vi "Logging Message Loop.vi"(8 "error in (no error)":errorcluster, 11 "Message Queues":T5) -> (0 "error out":errorcluster)   [LabVIEW 2018, in "Logging.lvlib"]
doc: "The message loop subVI to handle messages pertaining to logging data."
uses:
  Logging.lvlib
  Support/Message Queue/All Message Queues.ctl
  Support/Message Queue/Message Cluster.ctl
  Controls/Data Queue.ctl
  Controls/Acquired Data.ctl
  Controls/Data Notifier.ctl
  Settings/Settings.ctl
  Acquisition/Hardware Configuration.ctl
  Logging Configuration.ctl
  <vilib>/addons/database/Connection.llb/Conn ObjectReference.ctl
  Controls/Location Ring.ctl
  Controls/Time Remaining.ctl
  Logging State.ctl
  Support/Message Queue/Enqueue Message (Single).vi
  <vilib>/Utility/error.llb/Error Cluster From Error Code.vi
  <vilib>/ErrorRing/Error Ring.xnode
  support/Message Queue/Message Queue.lvlib
  <vilib>/addons/database/NI_Database_API.lvlib
  Acquisition/Acquisition.lvlib
  Settings/Settings.lvlib
panel:
  in  "C&C Data In":T1={"Hardware Configuration"={"COM Port"="", "Reference Distance"=0.0, "Sensor SN"=""}, "Logging Configuration"={"Log File Base Path"=path "", "Datafile Ref"=refnum, "Database Ref"=refnum}, "UI Refs"={"Start Ref"=refnum, "Settings Ref"=refnum, "Stop Ref"=refnum, "Exit Ref"=refnum, "Status Ref"=refnum, "Data Ref"=refnum, "StatusBox Ref"=refnum, "Location Ref"=refnum, "Operator Ref"=refnum, "Time Ref"=refnum, "Test in Progess Ref"=refnum}, "Calibration Data"={"calibrationID"=0, "operatorID"=0, "sensorID"=0, "start_time"="", "end_time"="", "offset"=0.0, "offset_units"="", "ring_time"=0.0, "error"=0.0, "Passed"=0, "data_storage_location"="", "comments"=""}, "Time Elapsed"=0, "Samples Required"=480} {"Hardware Configuration"."Reference Distance" format="%.3g"}
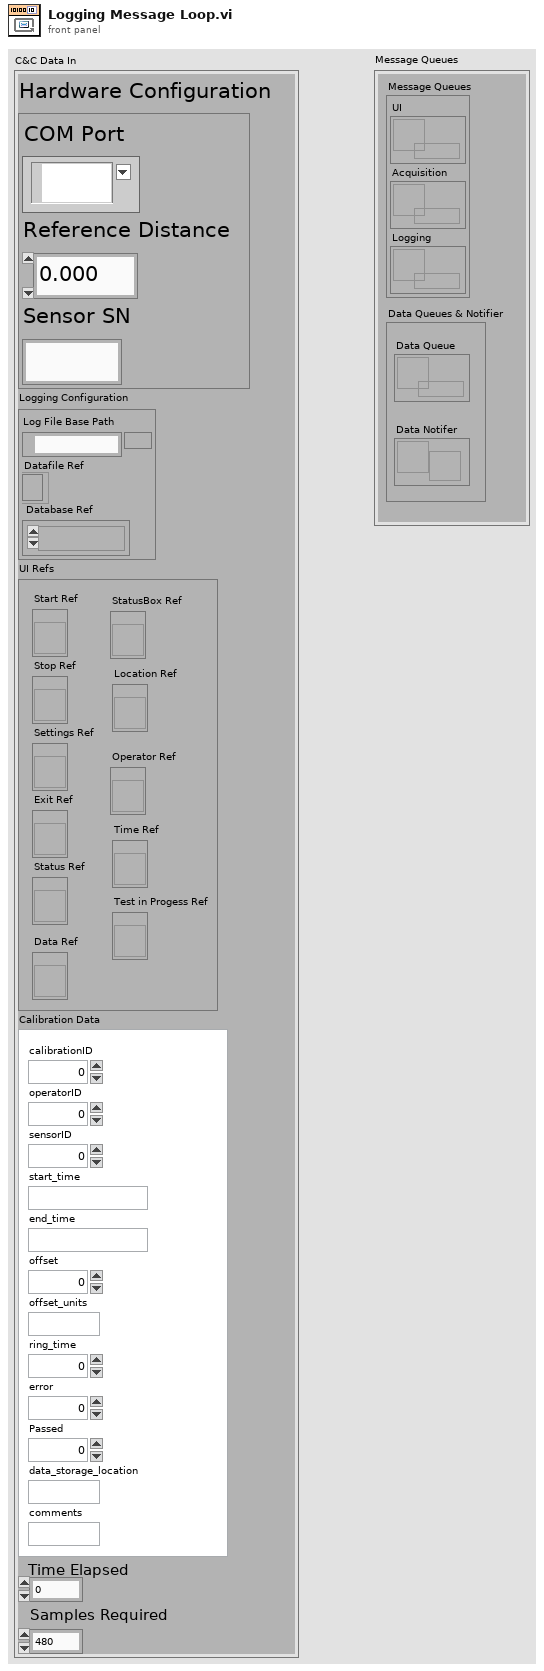
[diagram p1: front panel]
types:
  T1 = typedef "Settings.lvlib/Settings.ctl" = cluster{"Hardware Configuration":T2, "Logging Configuration":T3, "UI Refs":cluster{"Start Ref":refnum<vi>, "Settings Ref":refnum<vi>, "Stop Ref":refnum<vi>, "Exit Ref":refnum<vi>, "Status Ref":refnum<vi>, "Data Ref":refnum<vi>, "StatusBox Ref":refnum<vi>, "Location Ref":refnum<vi>, "Operator Ref":refnum<vi>, "Time Ref":refnum<vi>, "Test in Progess Ref":refnum<vi>}, "Calibration Data":cluster{"calibrationID":u16, "operatorID":u16, "sensorID":u16, "start_time":string, "end_time":string, "offset":dbl, "offset_units":string, "ring_time":dbl, "error":dbl, "Passed":u8, "data_storage_location":string, "comments":string}, "Time Elapsed":u16, "Samples Required":u16}
  T2 = typedef "Acquisition.lvlib/Hardware Configuration.ctl" = cluster{"COM Port":refnum<visa-resource-name>, "Reference Distance":dbl, "Sensor SN":string}
  T3 = typedef "Logging.lvlib/Logging Configuration.ctl" = cluster{"Log File Base Path":path, "Datafile Ref":refnum<file>, "Database Ref":T4}
  T4 = typedef "NI_Database_API.lvlib/Conn ObjectReference.ctl" = refnum<k1>
  T5 = typedef "Message Queue.lvlib/All Message Queues.ctl" = cluster{"Message Queues":cluster{"UI":refnum<queue>, "Acquisition":refnum<queue>, "Logging":refnum<queue>}, "Data Queues & Notifier":cluster{"Data Queue":T6, "Data Notifer":T7}}
  T6 = typedef "Data Queue.ctl" = refnum<queue>
  T7 = typedef "Data Notifier.ctl" = refnum<notifier>
  T8 = enum16{"open", "replace", "create", "open or create", "replace or create", "replace or create with confirmation"}
  T9 = typedef "Logging.lvlib/Logging State.ctl" = enum16{"Idle", "Logging"}
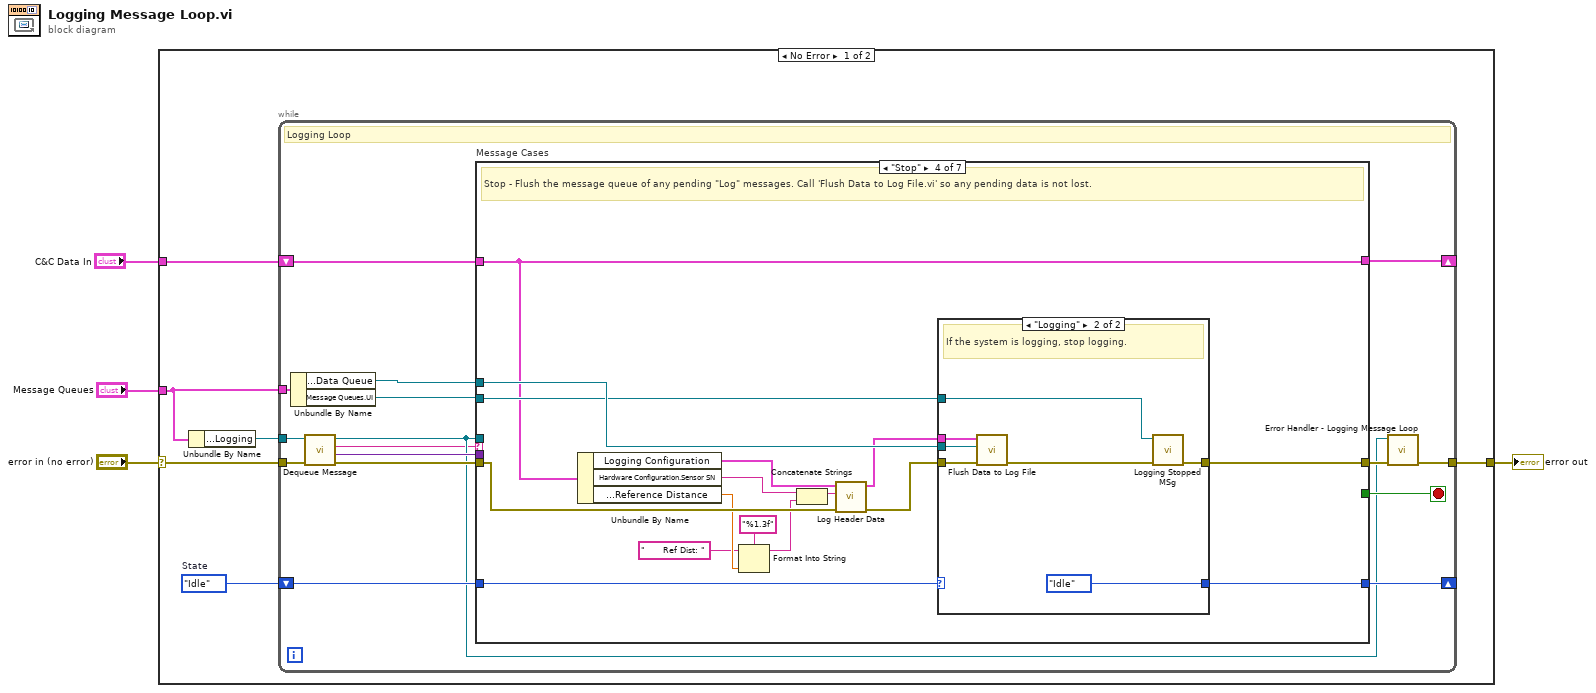
[diagram p0: block diagram]
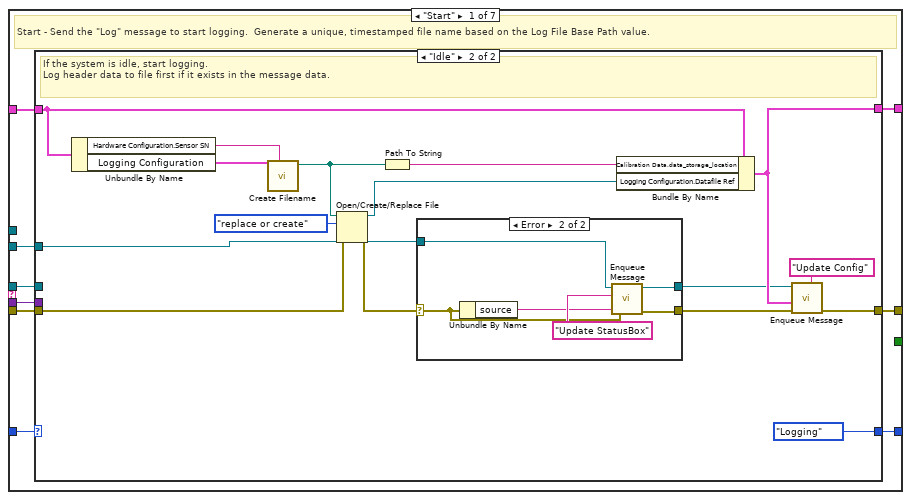
[diagram p2: hidden frame]
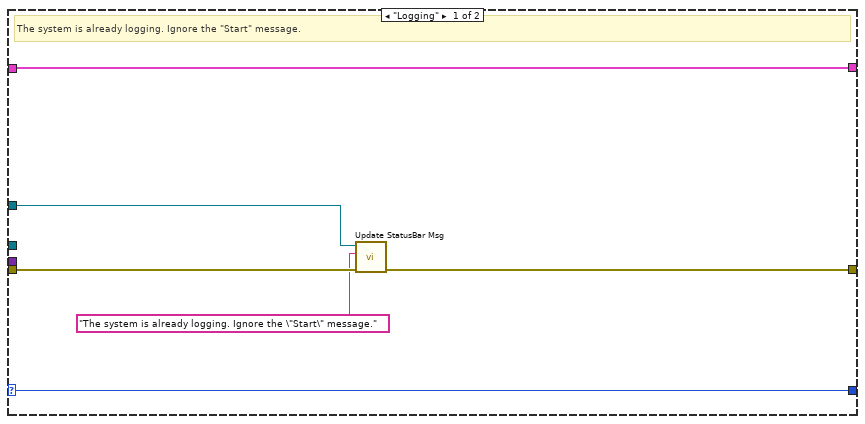
[diagram p3: hidden frame]
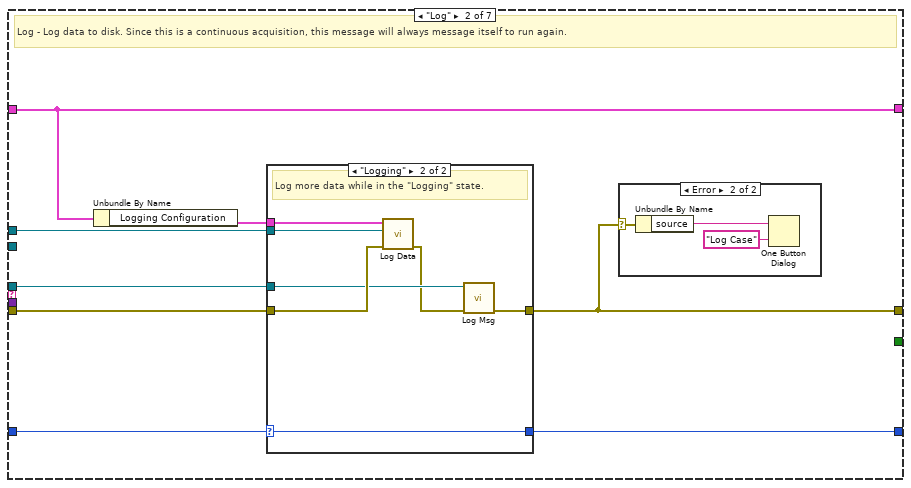
[diagram p5: hidden frame]
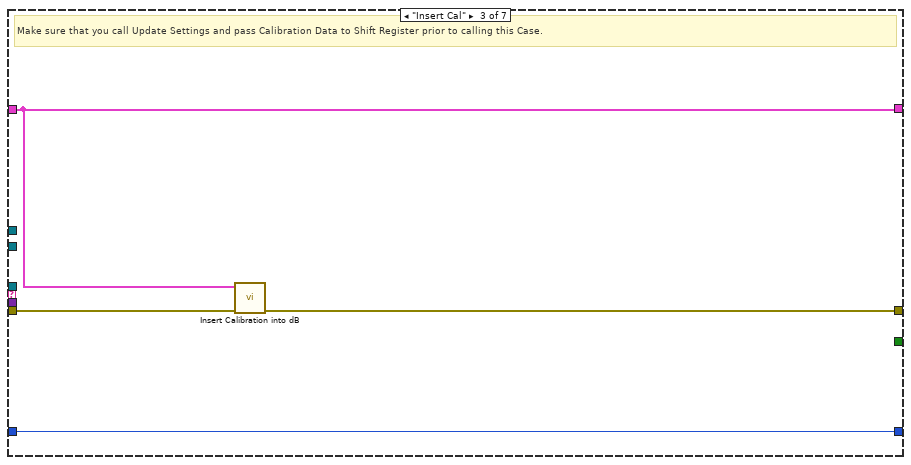
[diagram p8: hidden frame]
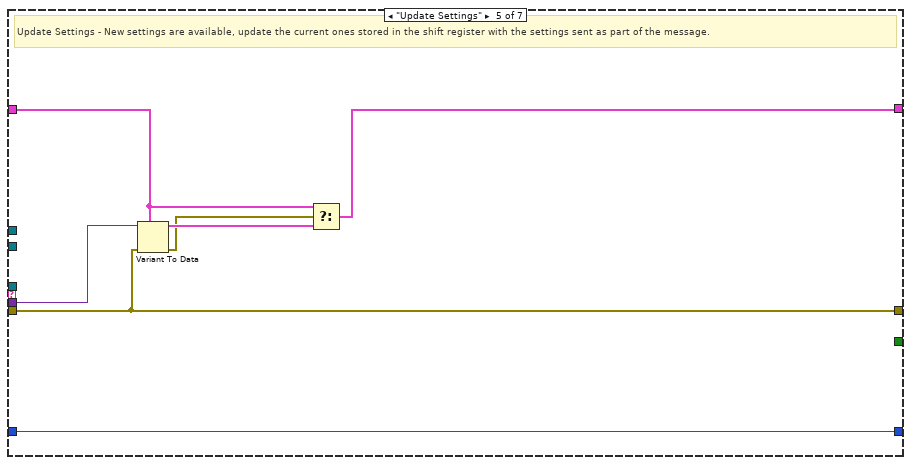
[diagram p10: hidden frame]
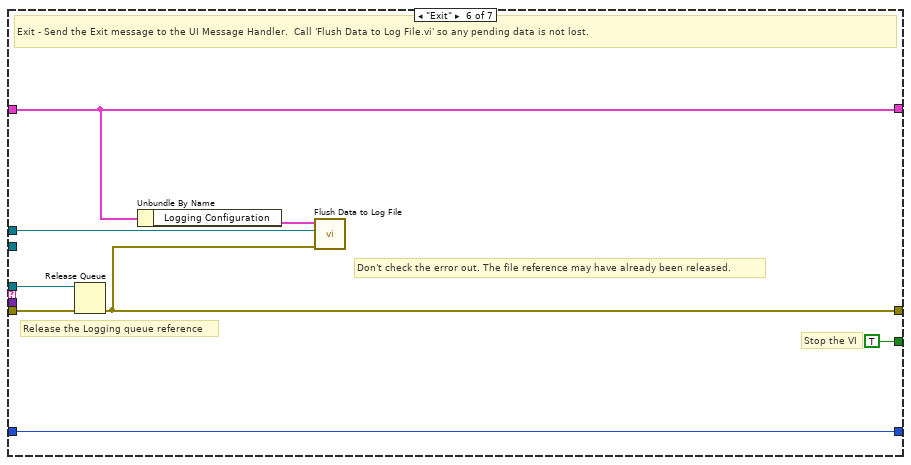
[diagram p11: hidden frame]
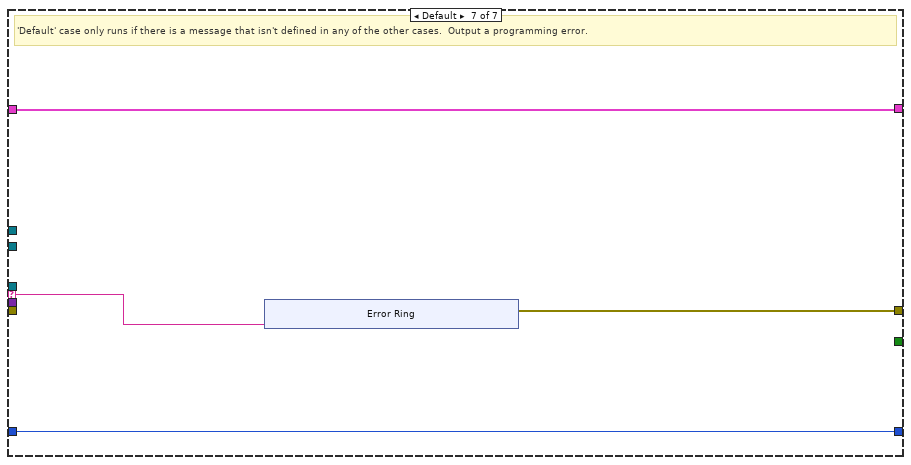
[diagram p12: hidden frame]
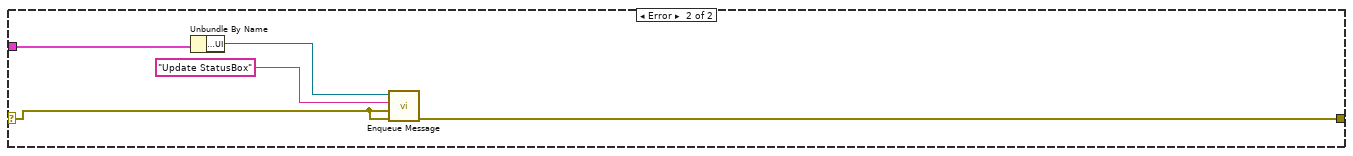
[diagram p13: hidden frame]
diagram:
  n1 = case shown="No Error" "error in (no error)" {
    selector: "error in (no error)" -> [w8 w141]
    tunnel: "Message Queues" -> [w6 w145]
    tunnel: [w9 w142] -> w3
    tunnel: "C&C Data In" -> [w5 _]
    frame No Error {
      w7 = Logging_State."Idle"  # State
      n2 = Unbundle By Name(w6) -> ("Message Queues.Logging"=w10:refnum<queue>)
      n3 = while {
        tunnel: w10 -> [w15]
        shift-right: [w21] -> _
        shift-left: w7 -> [w22]
        tunnel: w8 -> [w25]
        tunnel: [w20] -> w9
        tunnel: w6 -> [w18]
        shift-right: [w11] -> _
        shift-left: w5 -> [w12]
        stop <- w26 stop-if-true
        # "Logging Loop"
        n4 = Unbundle By Name(w18) -> ("Data Queues & Notifier.Data Queue"=w17:T6, "Message Queues.UI"=w16:refnum<queue>)
        n5 = call "Dequeue Message.vi"("error in (no error)"=w25, "Message Queue"=w15) -> ("error out"=w24:errorcluster, "Message Data"=w23:variant, "Message"=w13:string, "dup Message Queue"=w14:refnum<queue>)  [unwired: 6 in]
        n6 = case "Message Cases" shown="\"Stop\"" w13 {
          selector: w13 -> [_ _ _ _ _ _ w131]
          tunnel: w14 -> [w34 w73 _ _ _ w127 _]
          tunnel: w24 -> [w33 w72 w88 w96 w119 w128 _]
          tunnel: [w35 w66 w87 w105 w119 w126 w132] -> w19
          tunnel: [_ _ _ _ _ TRUE _] -> w26
          tunnel: w23 -> [w30 _ _ _ w121 _ _]
          tunnel: w16 -> [w29 _ _ w101 _ _ _]
          tunnel: w17 -> [_ w69 _ w104 _ w125 _]
          tunnel: w22 -> [w32 w71 w89 w103 w118 w124 w133]
          tunnel: [w31 w70 w89 w102 w118 w124 w133] -> w21
          tunnel: w12 -> [w28 w68 w86 w100 w117 w123 w130]
          tunnel: [w27 w68 w86 w100 w116 w123 w130] -> w11
          frame "Start" {
            # "Start - Send the \"Log\" message to start logging.  Generate a unique, timestamped file name based on the Log File Base Path value."
            n7 = case shown="\"Idle\"" w32 {
              selector: w32 -> [w41 _]
              tunnel: [w37 w48] -> w35
              tunnel: w34 -> [_ _]
              tunnel: w33 -> [w38 w55]
              tunnel: [w41 Logging_State."Logging" ("State")] -> w31
              tunnel: w30 -> [_ _]
              tunnel: w29 -> [w39 w47]
              tunnel: w28 -> [w40 w50]
              tunnel: [w40 w51] -> w27
              frame "Logging" {
                # "The system is already logging. Ignore the \"Start\" message."
                n8 = call "Update StatusBar Msg.vi"("error in (no error)"=w38, "Ready..."="The system is already logging. Ignore the \"Start\" message.", "Queue in"=w39) -> ("error out"=w37:errorcluster)  [unwired: 7 in, 1 out]
              }
              frame "Idle" {
                # "If the system is idle, start logging. \nLog header data to file first if it exists in the message data."
                n9 = Unbundle By Name(w50) -> ("Hardware Configuration.Sensor SN"=w42:string, "Logging Configuration"=w49:T3)
                n10 = call "Create Filename.vi"("Sensor SN"=w42, "Logging Configuration"=w49) -> ("appended path"=w53:path)  [unwired: 9 in]
                n11 = Open/Create/Replace File(file path (use dialog)=w53, error in=w55, operation (0:open)=T8."replace or create") -> (refnum out=w54:refnum<file>, error out=w45:errorcluster)  [unwired: 3 in, 1 out]
                n12 = Path To String(path=w53) -> (string=w43:string)
                n13 = case shown="Error" w45 {
                  selector: w45 -> [w59 w60]
                  tunnel: w47 -> [w58 w64]
                  tunnel: [w58 w63] -> w46
                  tunnel: [w59 w62] -> w44
                  frame No Error {
                  }
                  frame Error {
                    n14 = Unbundle By Name(w60) -> ("source"=w61:string)
                    n15 = call-poly "Enqueue Message.vi"("error in (no error)"=w60, "Message Data"=w61, "Message"="Update StatusBox", "Message Queue"=w64) -> ("error out"=w62:errorcluster, "dup Message Queue"=w63:refnum<queue>)  [unwired: 6 in]
                  }
                }
                n16 = Bundle By Name(cluster=w50, "Calibration Data.data_storage_location"=w43, "Logging Configuration.Datafile Ref"=w54) -> (w51:T1)
                n17 = call-poly "Enqueue Message.vi"("error in (no error)"=w44, "Message Data"=w51, "Message"="Update Config", "Message Queue"=w46) -> ("error out"=w48:errorcluster)  [unwired: 6 in, 1 out]
              }
            }
          }
          frame "Log" {
            # "Log - Log data to disk. Since this is a continuous acquisition, this message will always message itself to run again."
            n18 = Unbundle By Name(w68) -> ("Logging Configuration"=w67:T3)
            n19 = case shown="\"Logging\"" w71 {
              selector: w71 -> [w78 w84]
              tunnel: [w77 w79] -> w66
              tunnel: w73 -> [_ w81]
              tunnel: w69 -> [_ w85]
              tunnel: w72 -> [w77 w83]
              tunnel: w67 -> [_ w82]
              tunnel: [w78 w84] -> w70
              frame "Idle" {
                # "Ignore \"Log\" messages when the logging is idle."
              }
              frame "Logging" {
                # "Log more data while in the \"Logging\" state."
                n20 = call "Log Data.vi"("error in (no error)"=w83, "Data Queue"=w85, "Logging Configuration"=w82) -> ("error out"=w80:errorcluster)  [unwired: 8 in]
                n21 = call "Log Msg.vi"("error in (no error)"=w80, "Queue in"=w81) -> ("error out"=w79:errorcluster)  [unwired: 9 in]
              }
            }
            n22 = case shown="Error" w66 {
              selector: w66 -> [_ w75]
              frame No Error {
              }
              frame Error {
                n23 = Unbundle By Name(w75) -> ("source"=w76:string)
                n24 = One Button Dialog(message=w76, button name ("OK")="Log Case") -> ()  [unwired: 1 out]
              }
            }
          }
          frame "Insert Cal" {
            # "Make sure that you call Update Settings and pass Calibration Data to Shift Register prior to calling this Case."
            n25 = call "Insert Calibration into dB.vi"("error in (no error)"=w88, "C&C Data In"=w86) -> ("error out"=w87:errorcluster)  [unwired: 9 in]
          }
          frame "Stop" {
            # "Stop - Flush the message queue of any pending \"Log\" messages. Call 'Flush Data to Log File.vi' so any pending data is not lost."
            n26 = Unbundle By Name(w100) -> ("Logging Configuration"=w99:T3, "Hardware Configuration.Sensor SN"=w95:string, "Hardware Configuration.Reference Distance"=w94:dbl)
            n27 = Format Into String(format string="%1.3f", initial string="      Ref Dist: " ("format string"), w94) -> (resulting string=w91:string)  [unwired: 1 in, 1 out]
            n28 = Concatenate Strings(w95, w91) -> (w93:string)
            n29 = call "Log Header Data.vi"("error in (no error)"=w96, "Header Data"=w93, "Logging Configuration in"=w99) -> ("error out"=w97:errorcluster, "Logging Configuration out"=w98:T3)  [unwired: 7 in]
            n30 = case shown="\"Logging\"" w103 {
              selector: w103 -> [w106 _]
              tunnel: [w107 w110] -> w105
              tunnel: w104 -> [_ w113]
              tunnel: w97 -> [w107 w112]
              tunnel: [w106 Logging_State."Idle" ("State")] -> w102
              tunnel: w101 -> [_ w109]
              tunnel: w98 -> [_ w108]
              frame "Idle" {
                # "The system is already idle. Ignore the \"Stop\" message."
              }
              frame "Logging" {
                # "If the system is logging, stop logging."
                n31 = call "Flush Data to Log File.vi"("error in (no error)"=w112, "Data Queue"=w113, "Logging Configuration"=w108) -> ("error out"=w114:errorcluster)  [unwired: 8 in]
                n32 = call "Logging Stopped MSg.vi"("error in (no error)"=w114, "Queue in"=w109) -> ("error out"=w110:errorcluster)  [unwired: 9 in]
              }
            }
          }
          frame "Update Settings" {
            # "Update Settings - New settings are available, update the current ones stored in the shift register with the settings sent as part of the message."
            n33 = Variant To Data(error in=w119, type=w117, Variant=w121) -> (data=w120:T1, error out=w115:errorcluster)
            n34 = Select(t=w117, s=w115, f=w120) -> (s? t:f=w116:T1)
          }
          frame "Exit" {
            # "Don't check the error out. The file reference may have already been released."
            # "Release the Logging queue reference"
            # "Stop the VI"
            # "Exit - Send the Exit message to the UI Message Handler.  Call 'Flush Data to Log File.vi' so any pending data is not lost."
            n35 = Release Queue(queue=w127, error in (no error)=w128) -> (error out=w126:errorcluster)  [unwired: 1 in, 2 out]
            n36 = Unbundle By Name(w123) -> ("Logging Configuration"=w122:T3)
            n37 = call "Flush Data to Log File.vi"("error in (no error)"=w126, "Data Queue"=w125, "Logging Configuration"=w122) -> ()  [unwired: 8 in, 1 out]
          }
          frame Default {
            # "'Default' case only runs if there is a message that isn't defined in any of the other cases.  Output a programming error."
            n38 = xnode "Error Ring"("parameter 0"=w131) -> ("error out"=w132:errorcluster)
          }
        }
        n39 = call "Error Handler - Logging Message Loop.vi"("error in (no error)"=w19, "Message Queue"=w14) -> ("dup error in"=w20:errorcluster)  [unwired: 8 in, 1 out]
      }
    }
    frame Error {
      n40 = Unbundle By Name(w145) -> ("Message Queues.UI"=w143:refnum<queue>)
      n41 = call-poly "Enqueue Message.vi"("error in (no error)"=w141, "Message Data"=w141, "Message"="Update StatusBox", "Message Queue"=w143) -> ("error out"=w142:errorcluster)  [unwired: 6 in, 1 out]
    }
  }
  "error out" <- w3
